vi "ConvertVoltToDegree.vi"(10 "Tension":dbl) -> (2 "Température":dbl)   [LabVIEW 2022 SP3]
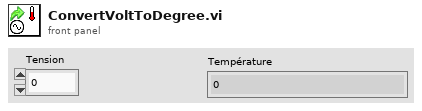
[diagram p1: front panel]
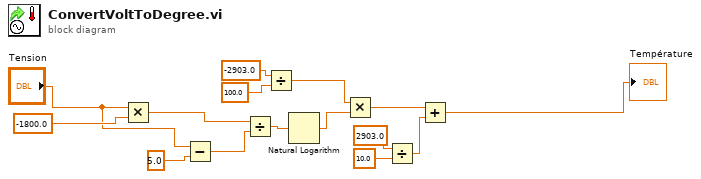
[diagram p0: block diagram]
diagram:
  n1 = Multiply(x="Tension", y=-1800.0) -> (x*y=w14:dbl)
  n2 = Subtract(x="Tension", y=5.0 ("x")) -> (x-y=w13:dbl)
  n3 = Divide(x=w14, y=w13) -> (x/y=w10:dbl)
  n4 = Divide(x=-2903.0, y=100.0) -> (x/y=w8:dbl)
  n5 = Natural Logarithm(1:w10) -> (0:w9:dbl)
  n6 = Multiply(x=w8, y=w9) -> (x*y=w7:dbl)
  n7 = Divide(x=2903.0, y=10.0) -> (x/y=w4:dbl)
  n8 = Add(x=w7, y=w4) -> (x+y=→"Température":dbl)
